vi "Parse Number.vi"(1 "String":string) -> (0 "Number":dbl)   [LabVIEW 2017, in "Apple script.lvlib"]
doc: "Parses a string to a number."
uses:
  Apple script.lvlib
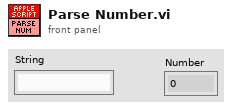
[diagram p1: front panel]
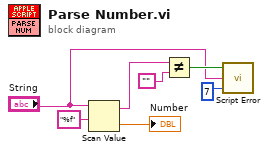
[diagram p0: block diagram]
diagram:
  n1 = Scan Value(string="String", format string="%f") -> (output string=w5:string, value=→"Number":dbl)  [unwired: 1 in]
  n2 = Not Equal?(x=w5, y="") -> (x != y?=w2:bool)
  n3 = call "Script Error.vi"("Error?"=w2, "Error Details"="String", "Error Code"=7) -> ()  [unwired: 2 in, 1 out]
